vi "Plane Fit.vi"(8 "Sensitivity":dbl=3.5, 9 "Z":dbl, 10 "Nano Z":dbl, 11 "X":dbl) -> (2 "Output":dbl, 3 "Clicks":dbl)   [LabVIEW 2019]
uses:
  <userlib>/HapticSTM/HapticSTM.lvlib
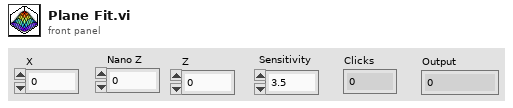
[diagram p1: front panel]
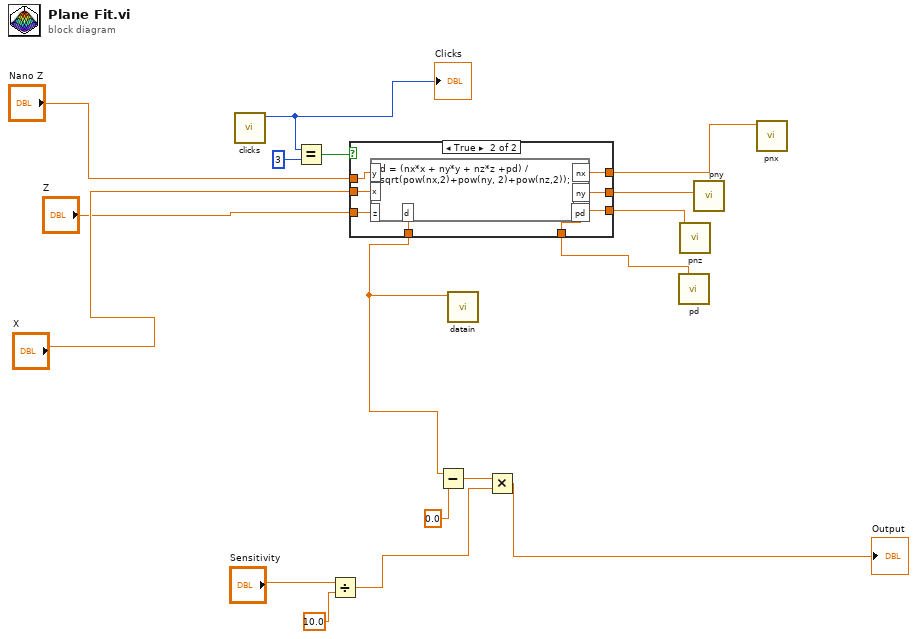
[diagram p0: block diagram]
diagram:
  n1 = call <userlib>:"clicks.vi"() -> ("function return"=w10:i32)  [unwired: 11 in]
  "Clicks" <- w10
  n2 = Equal?(x=w10, y=3) -> (x = y?=w8:bool)
  n3 = Divide(x="Sensitivity", y=10.0) -> (x/y=w16:dbl)
  n4 = call <userlib>:"pd.vi"() -> ("function return"=w11:dbl)  [unwired: 11 in]
  n5 = call <userlib>:"pnz.vi"() -> ("function return"=w12:dbl)  [unwired: 11 in]
  n6 = call <userlib>:"pny.vi"() -> ("function return"=w6:dbl)  [unwired: 11 in]
  n7 = call <userlib>:"pnx.vi"() -> ("function return"=w7:dbl)  [unwired: 11 in]
  n8 = case shown="True" w8 {
    tunnel: "X" -> [_ w26]
    tunnel: [w18 w25] -> w1
    tunnel: w7 -> [_ w24]
    tunnel: w6 -> [_ w23]
    tunnel: w12 -> [_ w22]
    tunnel: w11 -> [_ w21]
    tunnel: "Nano Z" -> [w18 w20]
    tunnel: "Z" -> [_ w19]
    frame False {
    }
    frame True {
      n9 = formula code="d = (nx*x + ny*y + nz*z +pd) / sqrt(pow(nx,2)+pow(ny, 2)+pow(nz,2));"("y"=w20, "z"=w19, "x"=w26, "nx"=w24, "ny"=w23, "nz"=w22, "pd"=w21) -> ("d"=w25:dbl)
    }
  }
  n10 = Subtract(x=w1, y=0.0 ("x")) -> (x-y=w17:dbl)
  n11 = call <userlib>:"datain.vi"("output"=w1) -> ()  [unwired: 11 in]
  n12 = Multiply(x=w17, y=w16) -> (x*y=→"Output":dbl)
